vi "03AMT800_RPMmeasure.vi"() -> ()   [LabVIEW 2017]
uses:
  <vilib>/Analysis/baseanly.llb/Mean (DBL).vi
  <vilib>/Utility/file.llb/Write Delimited Spreadsheet (DBL).vi
  <vilib>/Analysis/NI_AALBase.lvlib
panel:
  in  "stop":bool
  out "TIME":dbl format="%<%H:%M:%S>t"
  out "XY Graph":cluster{dbl[], dbl[]}(graph)
  out "SPM":dbl format="%0.2f"
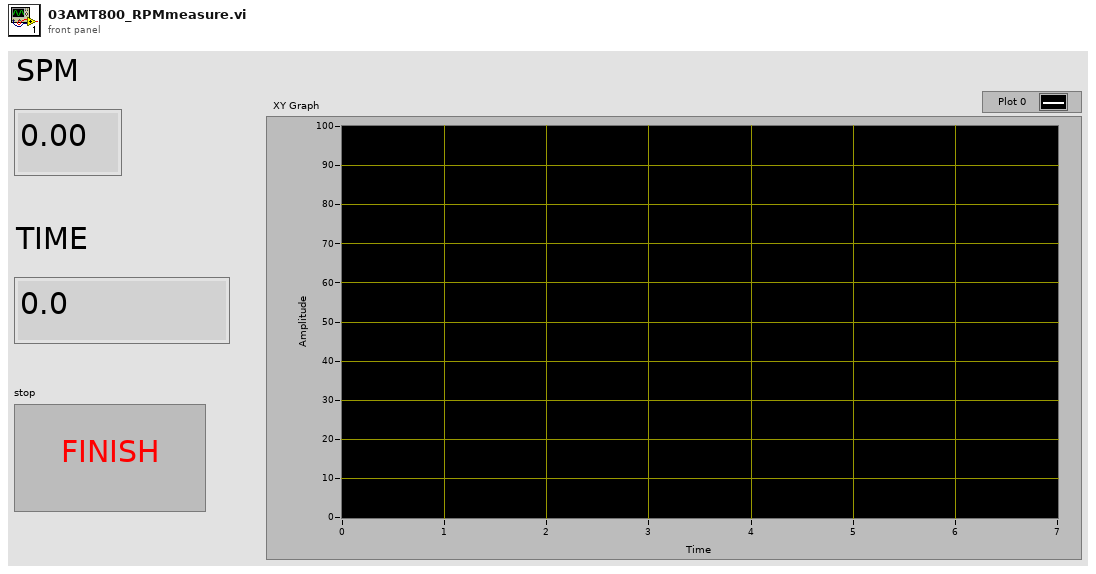
[diagram p1: front panel]
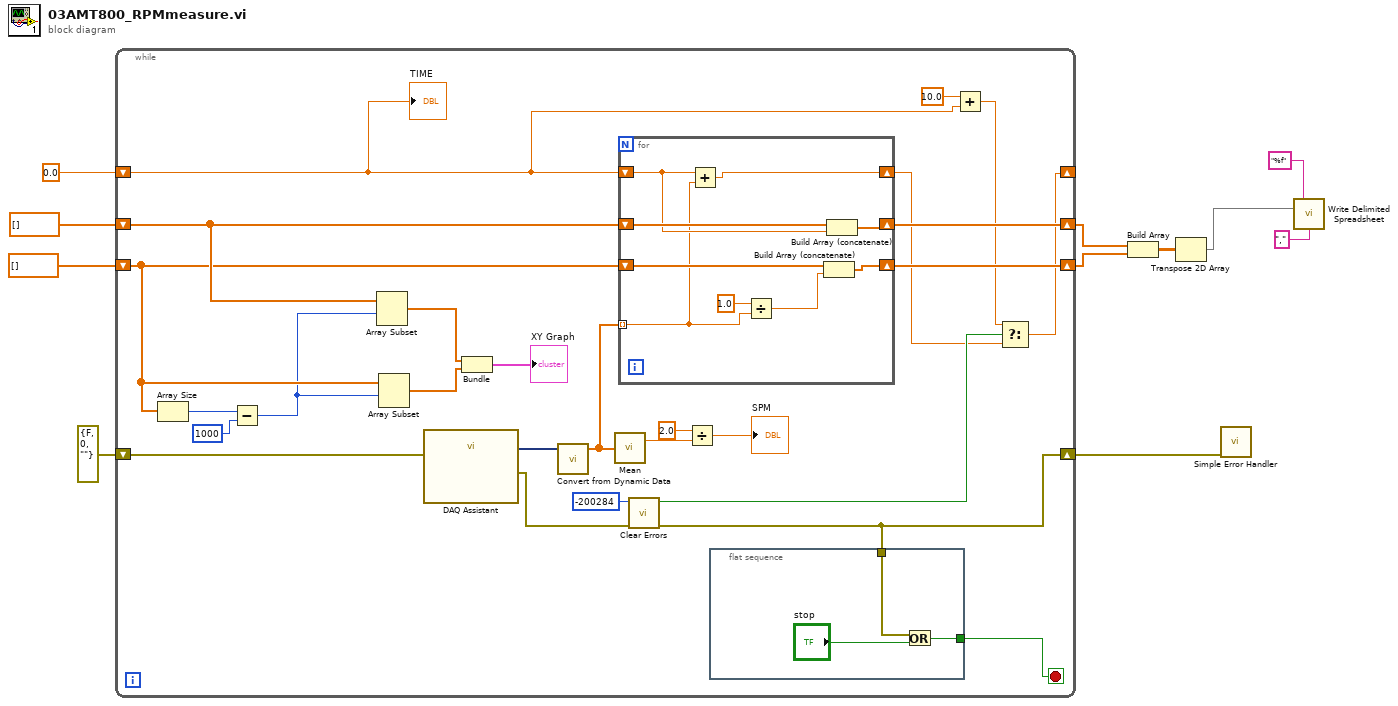
[diagram p0: block diagram]
diagram:
  n1 = while {
    shift-right: [w13] -> w1
    shift-left: errorcluster {"status"=FALSE, "code"=0, "source"=""} ("error out") -> [w37]
    shift-right: [w31] -> w7
    shift-left: dbl[] [] -> [w28]
    shift-right: [w17] -> _
    shift-left: 0.0 -> [w12]
    shift-right: [w30] -> w6
    shift-left: dbl[] [] -> [w25]
    stop <- w19 stop-if-true
    n2 = Array Size(array=w25) -> (size(s)=w24:i32)
    n3 = Subtract(x=w24, y=1000) -> (x-y=w22:i32)
    n4 = Array Subset(array=w28, index=w22) -> (w26:dbl[])  [unwired: 1 in]
    n5 = Array Subset(array=w25, index=w22) -> (w27:dbl[])  [unwired: 1 in]
    n6 = call "DAQ Assistant"("error in"=w37) -> ("data"=w36:dynamicdata, "error out"=w20:errorcluster)  [unwired: 15 in, 2 out]
    n7 = Bundle(w26, w27) -> (→"XY Graph":cluster{dbl[], dbl[]})  [unwired: 1 in]
    n8 = call "Convert from Dynamic Data"("Dynamic Data Type"=w36) -> ("Array"=w32:dbl[])  [unwired: 3 in]
    n9 = call-poly <vilib>:"Mean.vi"("X"=w32) -> ("mean"=w35:dbl)  [unwired: 1 out]
    n10 = for {
      tunnel: w32 -> [w43] mode=indexing
      shift-right: [w47] -> w31
      shift-left: w28 -> [w48]
      shift-right: [w49] -> w16
      shift-left: w12 -> [w46]
      shift-right: [w41] -> w30
      shift-left: w25 -> [w45]
      n11 = Add(x=w46, y=w43) -> (x+y=w49:dbl)
      n12 = Divide(x=1.0, y=w43) -> (x/y=w42:dbl)
      n13 = Build Array (concatenate)(w45, w42) -> (w41:dbl[])
      n14 = Build Array (concatenate)(w48, w46) -> (w47:dbl[])
    }
    n15 = call <vilib>:"Clear Errors.vi"("error in (no error)"=w20, "specific error code to clear (0: all)"=-200284) -> ("error out"=w13:errorcluster, "specific error cleared?"=w18:bool)  [unwired: 4 in]
    n16 = Divide(x=2.0, y=w35) -> (x/y=→"SPM":dbl)
    n17 = flat-sequence {
      tunnel: [w39] -> w19
      tunnel: w13 -> [w38]
      frame #0 {
        n18 = Or(x=w38, y="stop") -> (x .or. y?=w39:bool)
      }
    }
    n19 = Add(x=10.0, y=w12) -> (x+y=w14:dbl)
    n20 = Select(t=w14, s=w18, f=w16) -> (s? t:f=w17:dbl)
    "TIME" <- w12
  }
  n21 = Build Array(w7, w6) -> (w4:dbl[][])
  n22 = Transpose 2D Array(2D array=w4) -> (transposed array=w3:dbl[][])
  n23 = call <vilib>:"Simple Error Handler.vi"("error in (no error)"=w1) -> ()  [unwired: 4 in, 5 out]
  n24 = call-poly <vilib>:"Write Delimited Spreadsheet.vi"("format (%.3f)"="%f", "2D data"=w3, "delimiter (\\t)"="," ("delimiter (\\t)")) -> ()  [unwired: 11 in, 2 out]
